vi "Test select pages Reader.vi"() -> ()   [LabVIEW 2019, in "Exaprom PDF.lvlib"]
uses:
  Controls/Concatenate Controls/PDF file to concatenate.ctl
  Controls/General Controls/Create, open or close.ctl
  Exaprom PDF.lvlib
panel:
  in  "File and pages":T1={"Path"=path "", "Pages"="all", "Password"=""}
  out "error out":errorcluster
  out "NumberOfPages":i32
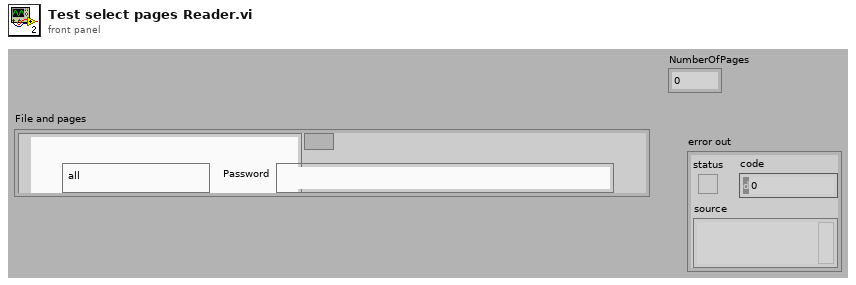
[diagram p1: front panel]
types:
  T1 = typedef "Exaprom PDF.lvlib/PDF file to concatenate.ctl" = cluster{"Path":path, "Pages":string, "Password":string}
  T2 = typedef "Exaprom PDF.lvlib/Create, open or close.ctl" = enum16{"Create", "Open", "Close"}
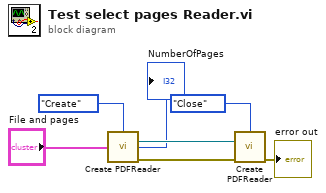
[diagram p0: block diagram]
diagram:
  n1 = call "Create PDFReader.vi"("Action"=Create,_open_or_close."Create", "File and pages"="File and pages") -> ("PdfReader OUT"=w4:refnum<k24>, "NumberOfPages"=→"NumberOfPages":i32, "error out"=w7:errorcluster)  [unwired: 10 in, 1 out]
  n2 = call "Create PDFReader.vi"("Action"=Create,_open_or_close."Close", "PdfReader IN"=w4, "error in (no error)"=w7) -> ("error out"=→"error out":errorcluster)  [unwired: 9 in, 3 out]
